vi "Enable Auto Channels.vi"(8 "error in (no error)":errorcluster, 11 "RemoteDataService in":refnum<class "RemoteDataService.lvclass">) -> (0 "error out":errorcluster, 3 "RemoteDataService out":refnum<class "RemoteDataService.lvclass">)   [LabVIEW 2020, in "Vecto.lvlib" / "RemoteDataService.lvclass"]
uses:
  RemoteDataService.lvclass
  RemoteDataService.lvclass/RemoteDataService.ctl
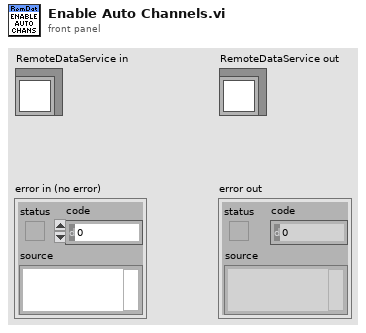
[diagram p1: front panel]
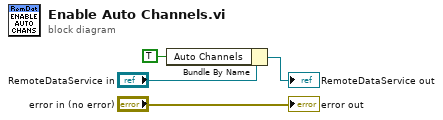
[diagram p0: block diagram]
diagram:
  n1 = Bundle By Name(cluster="RemoteDataService in", "Auto Channels"=TRUE) -> (→"RemoteDataService out":refnum<class "RemoteDataService.lvclass">)
  "error out" <- "error in (no error)"
